vi "TagBus_Get Tag Keys.vi"(10 "Tag Keys":string[](array[string])=["Load_kW", "EnergyStorage_kW", "Grid_kW"], 11 "TagBus":refnum<class "TagBus.lvclass">) -> (2 "Index Array":i32[](array[numeric]), 3 "TagBus out":refnum<class "TagBus.lvclass">)   [LabVIEW 2015, in "TagBus.lvclass"]
uses:
  TagBus.lvclass
  TagBus.lvclass/TagBus.ctl
  <vilib>/NI/Tag Bus/dictionary/data dictionary.lvclass
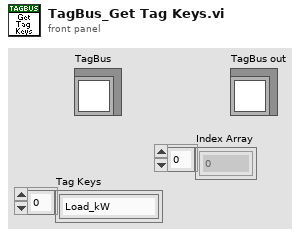
[diagram p1: front panel]
types:
  T1 = typedef "tag bus.lvlib/tag descriptor.lvclass/Data Type.ctl" = enum16{"Double", "Single", "I64", "I32", "I16", "I8", "U64", "U32", "U16", "U8", "Boolean", "String", "Array of Double", "Array of Single", "Array of I64", "Array of I32", "Array of I16", "Array of I8", "Array of U64", "Array of U32", "Array of U16", "Array of U8", "Array of Boolean", "Array of String"}
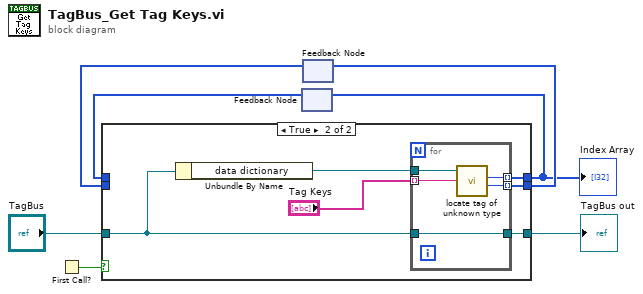
[diagram p0: block diagram]
diagram:
  n1 = First Call?() -> (First Call?: T/F=w4:bool)
  n2 = feedback #1() -> (w3:i32[])  [unwired: 1 in]
  n3 = feedback #2() -> (w7:T1[])  [unwired: 1 in]
  n4 = case shown="True" w4 {
    tunnel: "TagBus" -> [w8 w11]
    tunnel: [w10 w16] -> w5
    tunnel: w3 -> [w10 _]
    tunnel: [w9 w15] -> w6
    tunnel: w7 -> [w9 _]
    tunnel: [w8 w12] -> w1
    frame False {
    }
    frame True {
      n5 = Unbundle By Name(w11) -> ("data dictionary"=w13:refnum<class "data dictionary.lvclass">)
      n6 = for {
        tunnel: w13 -> [w21]
        tunnel: "Tag Keys" -> [w20] mode=indexing
        tunnel: [w19] -> w16 mode=indexing
        tunnel: [w18] -> w15 mode=indexing
        tunnel: [w17] -> w12
        tunnel: w11 -> [w17]
        n7 = call <vilib>:"locate tag of unknown type.vi"("name"=w20, "data dictionary in"=w21) -> ("data type"=w18:T1, "index"=w19:i32)  [unwired: 6 in, 2 out]
      }
    }
  }
  "Index Array" <- w5
  "TagBus out" <- w1
  n8 = feedback-in #1(w5) -> ()
  n9 = feedback-in #2(w6) -> ()
